vi "Format HV.vi"(4 "WorkTable":refnum<class "WorkTable Class.lvclass">, 6 "HV Points":T1[](array[typedef]), 8 "error in":errorcluster, 9 "Slot":i32, 10 "Chuck":i32, 11 "Console Log in":refnum<class "Console Log.lvclass">) -> (0 "error out":errorcluster, 2 "Formatted Address Pads":string[](array[string]), 3 "Console Log out":refnum<class "Console Log.lvclass">)   [LabVIEW 2011, in "Console Log.lvclass"]
uses:
  Console Log.lvclass
  Shared Components/WorkTable Class/WorkTable Class.lvclass
  Shared Components/Utils/Type Definitions/3d Point.ctl
  Shared Components/Vec3d Class/Vec3d Class.lvclass
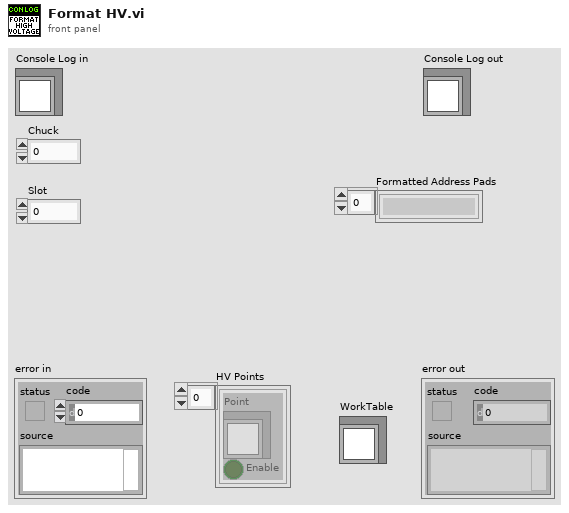
[diagram p1: front panel]
types:
  T1 = typedef "3d Point.ctl" = cluster{"Point":refnum<class "Vec3d Class.lvclass">, "Enable":bool}
  T2 = typedef "Worktable_Module Slot.ctl" = cluster{"Slot State":enum16{"Empty", "Unglued", "Stamped", "PartOnTop", "Weighted", "Unpotted", "Potted"}, "BBM Type":enum16{"None", "BBM", "GlassSlide"}, "HDI Type":enum16{"None", "HDI", "Polyimide"}, "Vacuum Channel":u8, "Location/Orientation BBM":T3, "Location/Orientation HDI":T3, "S/N":string}
  T3 = typedef "Position_Orientation.ctl" = cluster{"Center":refnum<class "Vec3d Class.lvclass">, "Orientation":refnum<class "Orient3d Class.lvclass">}
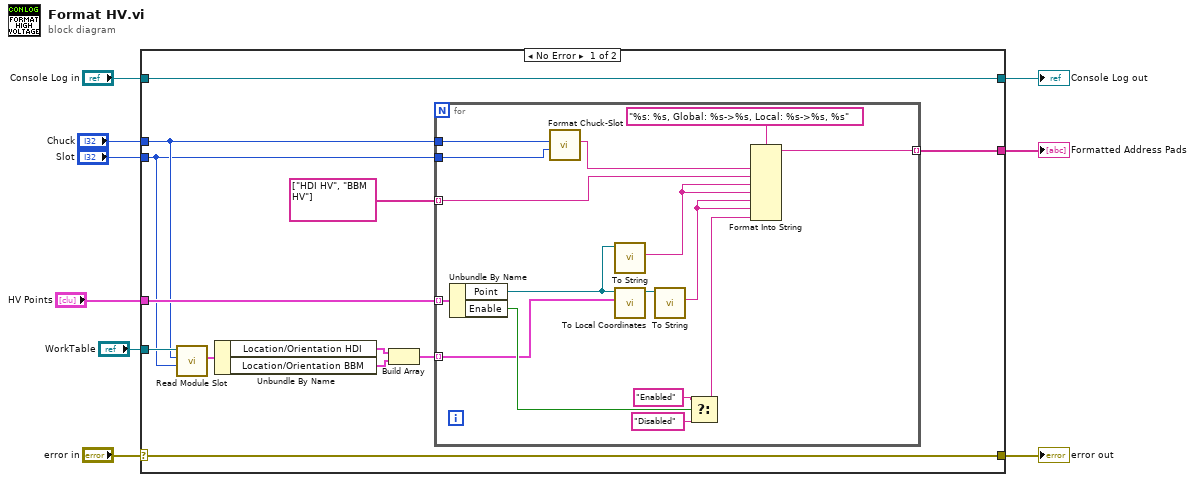
[diagram p0: block diagram]
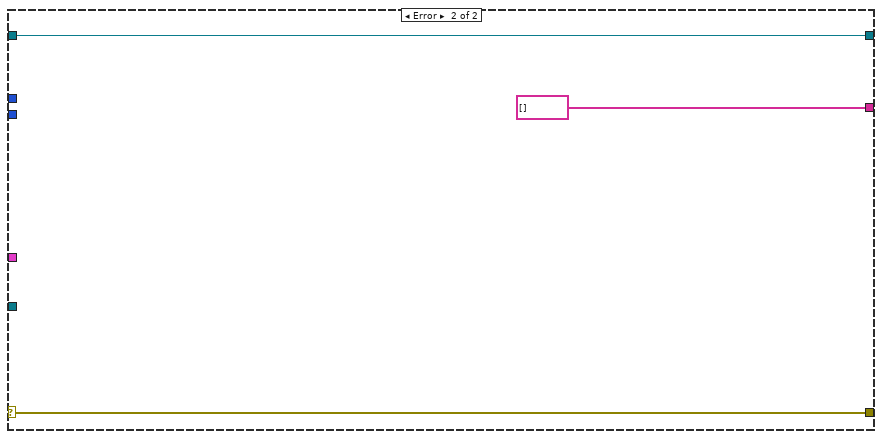
[diagram p2: hidden frame]
diagram:
  n1 = case shown="No Error" "error in" {
    selector: "error in" -> [w20 w40]
    tunnel: [w20 w40] -> w8
    tunnel: [w21 w39] -> w6
    tunnel: "Console Log in" -> [w21 w39]
    tunnel: "HV Points" -> [w19 _]
    tunnel: [w18 string[] []] -> w5
    tunnel: "Chuck" -> [w15 _]
    tunnel: "Slot" -> [w14 _]
    tunnel: "WorkTable" -> [w16 _]
    frame No Error {
      n2 = call-dynamic "Read Module Slot.vi"("slot"=w14, "chuck"=w15, "WorkTable in"=w16) -> ("Module Slot"=w13:T2)  [unwired: 6 in, 2 out]
      n3 = Unbundle By Name(w13) -> ("Location/Orientation HDI"=w11:T3, "Location/Orientation BBM"=w12:T3)
      n4 = Build Array(w11, w12) -> (w10:T3[])
      n5 = for {
        tunnel: w19 -> [w37] mode=indexing
        tunnel: [w32] -> w18 mode=indexing
        tunnel: string[] ["HDI HV", "BBM HV"] -> [w31] mode=indexing
        tunnel: w15 -> [w28]
        tunnel: w14 -> [w27]
        tunnel: w10 -> [w24] mode=indexing
        n6 = Unbundle By Name(w37) -> ("Point"=w25:refnum<class "Vec3d Class.lvclass">, "Enable"=w36:bool)
        n7 = call "Format Chuck-Slot.vi"("Slot"=w27, "Chuck"=w28) -> ("Formatted Chuck/Slot"=w30:string)  [unwired: 7 in, 2 out]
        n8 = call "To String.vi"("Vec3d in"=w25) -> ("Vec3d String"=w23:string)  [unwired: 8 in, 2 out]
        n9 = call "To Local Coordinates.vi"("Center/Orientation"=w24, "Global Coordinates"=w25) -> ("Local Coordinates"=w26:refnum<class "Vec3d Class.lvclass">)  [unwired: 8 in, 1 out]
        n10 = call "To String.vi"("Vec3d in"=w26) -> ("Vec3d String"=w22:string)  [unwired: 8 in, 2 out]
        n11 = Select(t="Enabled", s=w36, f="Disabled") -> (s? t:f=w29:string)
        n12 = Format Into String(format string="%s: %s, Global: %s->%s, Local: %s->%s, %s", w30, w31, w23, w23, w22, w22, w29) -> (resulting string=w32:string)  [unwired: 2 in, 1 out]
      }
    }
    frame Error {
    }
  }
  "error out" <- w8
  "Console Log out" <- w6
  "Formatted Address Pads" <- w5
